vi "Auto range.vi"(8 "error in (no error)":errorcluster, 10 "Auto Ranging?":T1=enum."On", 11 "VISA resource name":refnum<visa-resource-name>="GPIB0::21::INSTR") -> (0 "error out":errorcluster, 3 "VISA resource name out":refnum<visa-resource-name>)   [LabVIEW 2017]
uses:
  Auto Range control.ctl
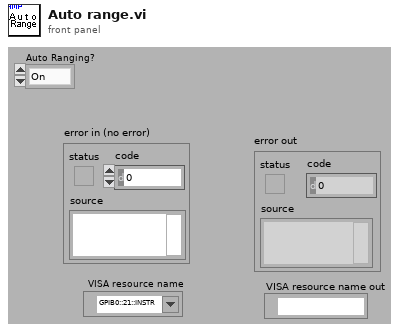
[diagram p1: front panel]
types:
  T1 = typedef "Auto Range control.ctl" = enum16{"Off", "On"}
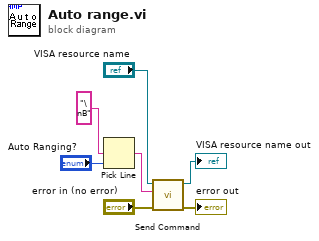
[diagram p0: block diagram]
diagram:
  n1 = Pick Line(multi-line string="\nB", line index="Auto Ranging?") -> (output string=w1:string)  [unwired: 1 in]
  n2 = call "Send Command.vi"("error in (no error)"="error in (no error)", "write buffer"=w1, "VISA resource name"="VISA resource name") -> ("error out"=→"error out":errorcluster, "VISA resource name out"=→"VISA resource name out":refnum<visa-resource-name>)  [unwired: 7 in]
